vi "10.7(navragen).vi"() -> ()   [LabVIEW 2019]
panel:
  out "Array":dbl[](array[numeric])
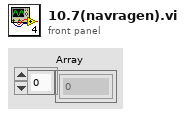
[diagram p1: front panel]
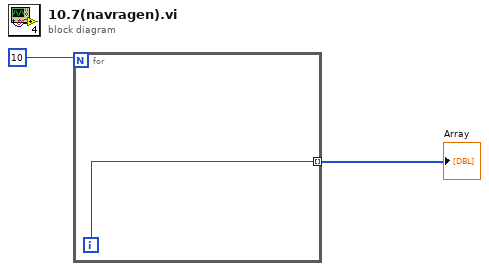
[diagram p0: block diagram]
diagram:
  n1 = for {
    N: 10 -> [_]
    tunnel: [w3] -> w1 mode=indexing
    i -> [w3]
  }
  "Array" <- w1
